vi "Skip schedule.vi"(8 "error in (no error)":errorcluster, 11 "Run Block in":refnum<class "Run Block.lvclass">) -> (0 "error out":errorcluster, 3 "Run Block out":refnum<class "Run Block.lvclass">)   [LabVIEW 2020, in "Run Utilities.lvlib" / "Run Block.lvclass"]
doc: "Moves current RUN and all scripts from the schedule to skipped RUNs"
uses:
  Run Block.lvclass
  Schedule/Schedule.lvclass
  Run Block.lvclass/Run Block.ctl
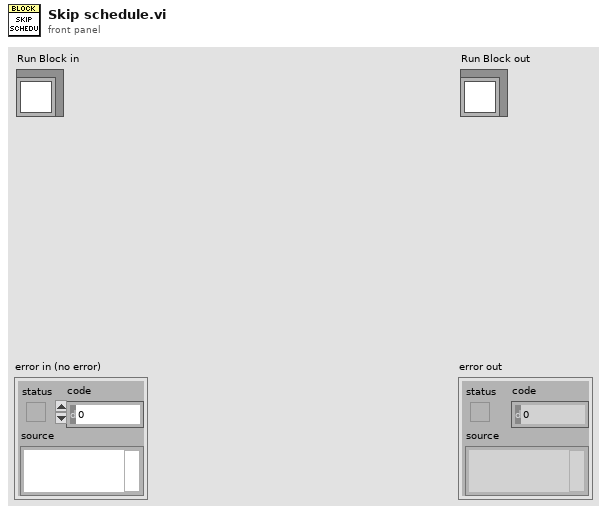
[diagram p1: front panel]
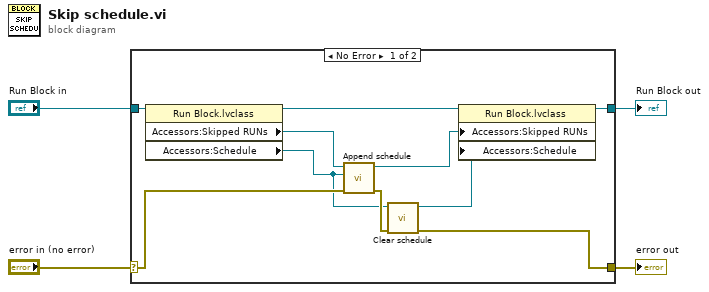
[diagram p0: block diagram]
diagram:
  n1 = case shown="No Error" "error in (no error)" {
    selector: "error in (no error)" -> [w14 w16]
    tunnel: [w6 w16] -> w3
    tunnel: [w11 w15] -> w1
    tunnel: "Run Block in" -> [w13 w15]
    frame No Error {
      n2 = property class="Run Block.lvclass"(reference=w13) -> (reference out=w12:refnum<class "Run Block.lvclass">, "Accessors:Skipped RUNs"=w10:refnum<class "Schedule.lvclass">, "Accessors:Schedule"=w5:refnum<class "Schedule.lvclass">)  [unwired: 1 in, 1 out]
      n3 = call-dynamic "Append schedule.vi"("error in (no error)"=w14, "Schedule to append"=w5, "Schedule in"=w10) -> ("error out"=w8:errorcluster, "Schedule out"=w9:refnum<class "Schedule.lvclass">)  [unwired: 7 in]
      n4 = call-dynamic "Clear schedule.vi"("error in (no error)"=w8, "Schedule in"=w5) -> ("error out"=w6:errorcluster, "Schedule out"=w7:refnum<class "Schedule.lvclass">)  [unwired: 8 in]
      n5 = property class="Run Block.lvclass"(reference=w12, "Accessors:Skipped RUNs"=w9, "Accessors:Schedule"=w7) -> (reference out=w11:refnum<class "Run Block.lvclass">)  [unwired: 1 in, 1 out]
    }
    frame Error {
    }
  }
  "error out" <- w3
  "Run Block out" <- w1
